vi "ConfigureBarPlot.vi"(0 "reference in":refnum<class "HTMLPlot.lvclass">, 5 "error in (no error)":errorcluster) -> (14 "reference out":refnum<class "HTMLPlot.lvclass">, 16 "fullHTML":string, 19 "error out":errorcluster)   [LabVIEW 2019, in "HTMLPlot.lvclass"]
uses:
  HTMLPlot.lvclass
panel:
  out "plotOptions":string
  out "plotData":string
  out "plotType":string
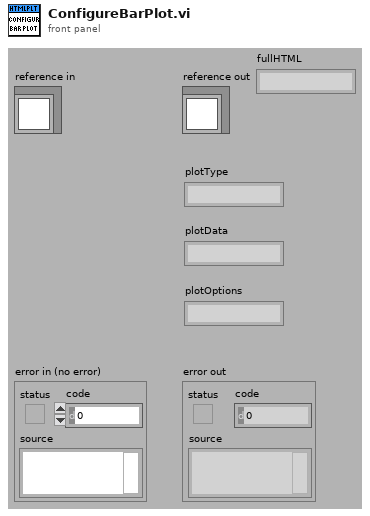
[diagram p1: front panel]
types:
  T1 = typedef "HTMLPlot.lvclass/ObjectAttributes.ctl" = cluster{"Attribute1":dbl, "GraphContainer":refnum<k7>, "ChartScriptFile":string, "UtilScriptFile(demoData)":string, "BaseHTML":string, "GenericProperties":cluster{"PlotType":T2, "PlotTitle":string, "XLabel":string, "YLabel":string, "ShowToolTip":bool}, "LegendProperties":cluster{"Show":bool, "Position":T3}, "BarPlot":cluster{"Dataset":dbl[][], "DatasetLabels":string[], "XLabels":string[], "PlotColours":u32[], "Stacked":bool}, "PiePlot":cluster{"Dataset":dbl[][], "DatasetLabels":string[], "PlotColours":u32[], "DoughnutStyle":bool, "PlotLabels":string[]}, "connection ID":refnum<k5>, "PortID":u64}
  T2 = typedef "HTMLPlot.lvclass/PlotType.ctl" = enum16{"bar", "line", "pie"}
  T3 = typedef "HTMLPlot.lvclass/LegendPosition.ctl" = enum16{"top", "right", "left", "bottom"}
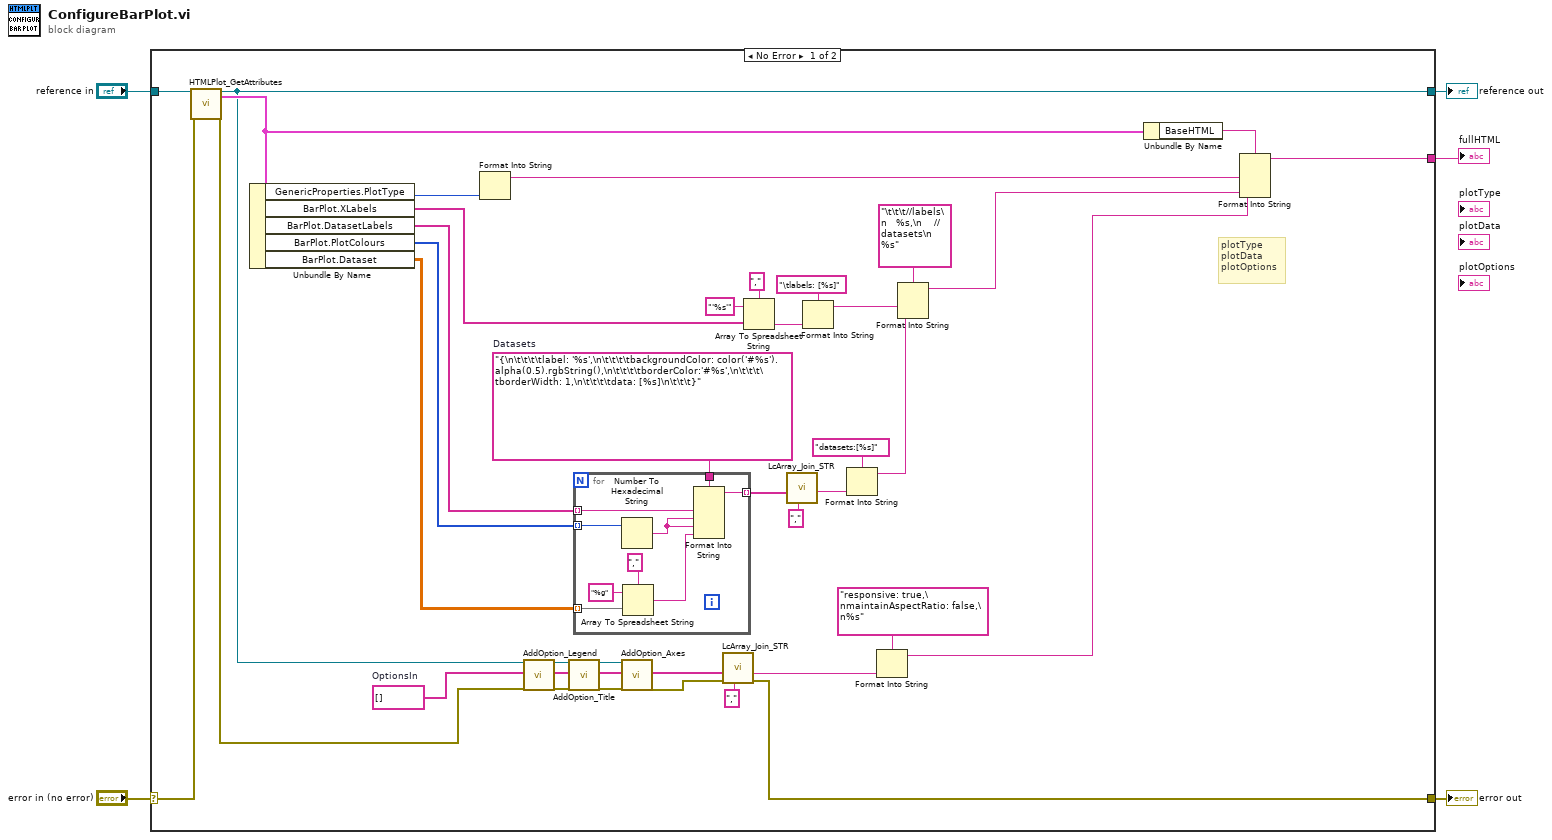
[diagram p0: block diagram]
diagram:
  n1 = case shown="No Error" "error in (no error)" {
    selector: "error in (no error)" -> [w45 w56]
    tunnel: [w13 w56] -> w4
    tunnel: [w10 w55] -> w2
    tunnel: "reference in" -> [w44 w55]
    tunnel: [w12 _] -> w1
    frame No Error {
      w23 = "{\n\t\t\t\tlabel: '%s',\n\t\t\t\tbackgroundColor: color('#%s').alpha(0.5).rgbString(),\n\t\t\t\tborderColor:'#%s',\n\t\t\t\tborderWidth: 1,\n\t\t\t\tdata: [%s]\n\t\t\t}"  # Datasets
      w11 = string[] []  # OptionsIn
      # "plotType\nplotData\nplotOptions"
      n2 = call "HTMLPlot_GetAttributes.vi"("reference in"=w44, "error in (no error)"=w45) -> ("reference out"=w10:refnum<class "HTMLPlot.lvclass">, "Data"=w19:T1, "error out"=w9:errorcluster)  [unwired: 14 in, 1 out]
      n3 = Unbundle By Name(w19) -> ("GenericProperties.PlotType"=w18:T2, "BarPlot.XLabels"=w35:string[], "BarPlot.DatasetLabels"=w36:string[], "BarPlot.PlotColours"=w37:u32[], "BarPlot.Dataset"=w15:dbl[][])
      n4 = Format Into String(w18) -> (resulting string=w17:string)  [unwired: 3 in, 1 out]
      n5 = call "AddOption_Legend.vi"("reference in"=w10, "OptionsIn"=w11, "error in (no error)"=w9) -> ("reference out"=w29:refnum<class "HTMLPlot.lvclass">, "OptionsOut"=w28:string[], "error out"=w27:errorcluster)  [unwired: 14 in]
      n6 = call "AddOption_Title.vi"("reference in"=w29, "OptionsIn"=w28, "error in (no error)"=w27) -> ("reference out"=w21:refnum<class "HTMLPlot.lvclass">, "OptionsOut"=w25:string[], "error out"=w20:errorcluster)  [unwired: 14 in]
      n7 = for {
        tunnel: w15 -> [w52] mode=indexing
        tunnel: w37 -> [w49] mode=indexing
        tunnel: w36 -> [w51] mode=indexing
        tunnel: [w47] -> w33 mode=indexing
        tunnel: w23 -> [w46]
        n8 = Number To Hexadecimal String(2:w49) -> (0:w48:string)  [unwired: 1 in]
        n9 = Array To Spreadsheet String(delimiter (Tab)=",", array=w52, 3:"%g" ("format string")) -> (spreadsheet string=w50:string)
        n10 = Format Into String(format string=w46, w51, w48, w48, w50) -> (resulting string=w47:string)  [unwired: 2 in, 1 out]
      }
      n11 = call "AddOption_Axes.vi"("reference in"=w21, "OptionsIn"=w25, "error in (no error)"=w20) -> ("OptionsOut"=w22:string[], "error out"=w14:errorcluster)  [unwired: 14 in, 1 out]
      n12 = call "LcArray_Join_STR.vi"("separator"=",", "error in (no error)"=w14, "Array"=w22) -> ("error out"=w13:errorcluster, "joined string"=w7:string)  [unwired: 7 in]
      n13 = Array To Spreadsheet String(delimiter (Tab)=",", array=w35, 3:"'%s'" ("format string")) -> (spreadsheet string=w38:string)
      n14 = call "LcArray_Join_STR.vi"("separator"=",", "Array"=w33) -> ("joined string"=w32:string)  [unwired: 8 in, 1 out]
      n15 = Format Into String(format string="\tlabels: [%s]", w38) -> (resulting string=w41:string)  [unwired: 2 in, 1 out]
      n16 = Format Into String(format string="datasets:[%s]", w32) -> (resulting string=w30:string)  [unwired: 2 in, 1 out]
      n17 = Format Into String(format string="responsive: true,\nmaintainAspectRatio: false,\n%s", w7) -> (resulting string=w6:string)  [unwired: 2 in, 1 out]
      n18 = Format Into String(format string="\t\t\t//labels\n   %s,\n    //datasets\n   %s", w41, w30) -> (resulting string=w16:string)  [unwired: 2 in, 1 out]
      n19 = Unbundle By Name(w19) -> ("BaseHTML"=w43:string)
      n20 = Format Into String(format string=w43, w17, w16, w6) -> (resulting string=w12:string)  [unwired: 2 in, 1 out]
    }
    frame Error {
    }
  }
  "error out" <- w4
  "reference out" <- w2
  "fullHTML" <- w1
